vi "Hormiga_analogWrite.vi"(8 "error in (no error)":errorcluster, 9 "Analog Value":u16(slide) scale=0.0..1000.0, 10 "Terminal":u8=13, 11 "VISA Refnum in":refnum<visa-resource-name>) -> (0 "error out":errorcluster, 2 "Returned Value":u16, 3 "VISA Refnum out":refnum<visa-resource-name>)   [LabVIEW 2016]
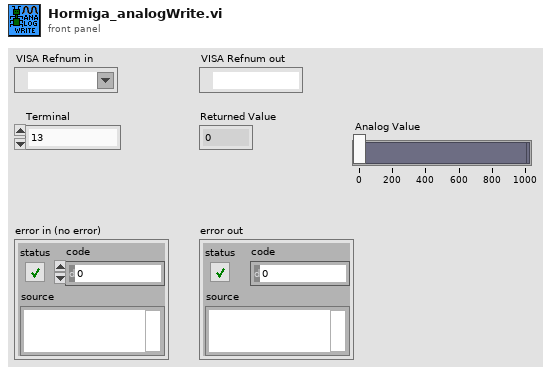
[diagram p1: front panel]
types:
  T1 = enum16{"pinMode", "digitalWrite", "digitalRead", "analogRead", "analogWrite"}
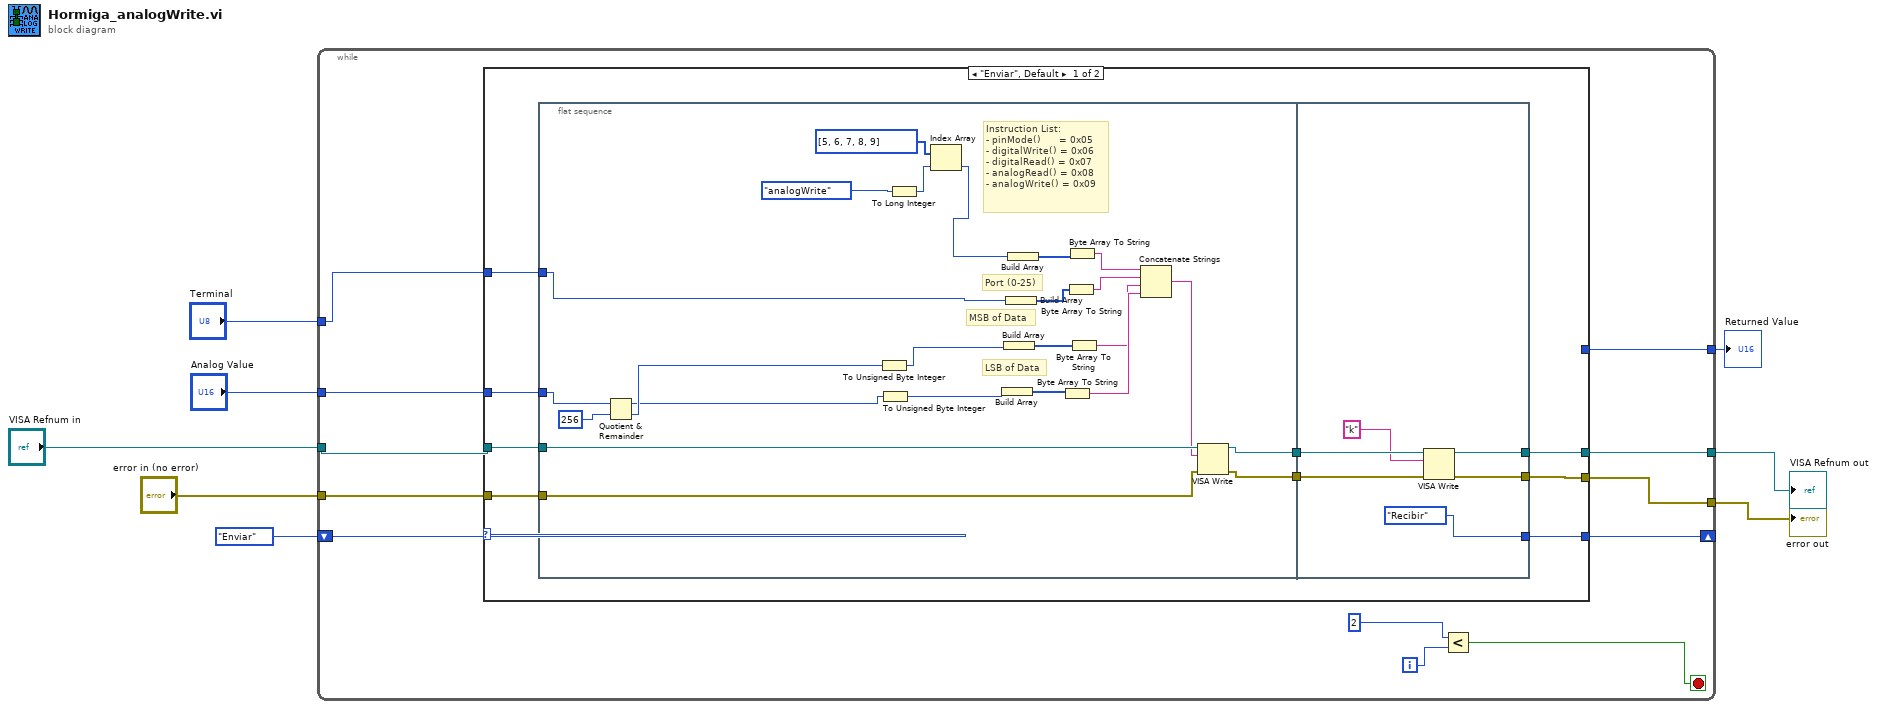
[diagram p0: block diagram]
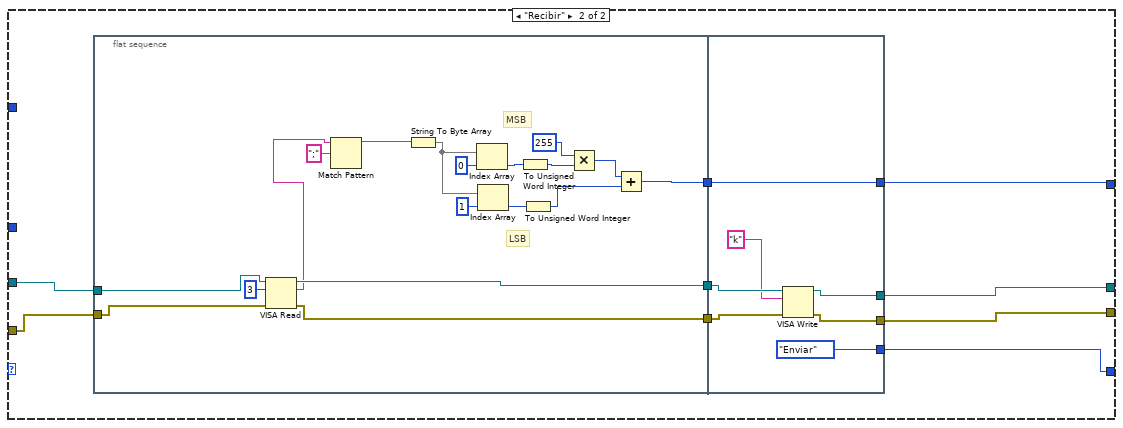
[diagram p2: hidden frame]
diagram:
  n1 = while {
    shift-right: [w15] -> _
    shift-left: enum16{"Enviar", "Recibir"}."Enviar" -> [w20]
    tunnel: "error in (no error)" -> [w19]
    tunnel: "VISA Refnum in" -> [w18]
    tunnel: [w17] -> w4
    tunnel: [w16] -> w5
    tunnel: "Terminal" -> [w11]
    tunnel: [w10] -> w8
    tunnel: "Analog Value" -> [w9]
    i -> [w13]
    stop <- w14 stop-if-true
    n2 = case shown="\"Enviar\", Default" w20 {
      tunnel: w19 -> [w29 w68]
      tunnel: w18 -> [w28 w67]
      tunnel: [w25 w64] -> w17
      tunnel: [w24 w63] -> w16
      tunnel: [w23 w62] -> w15
      tunnel: w11 -> [w22 _]
      tunnel: [_ w60] -> w10
      tunnel: w9 -> [w21 _]
      frame "Enviar", Default {
        n3 = flat-sequence {
          tunnel: w29 -> [w53]
          tunnel: w28 -> [w52]
          tunnel: [w51] -> w27
          tunnel: [w50] -> w26
          tunnel: w22 -> [w30]
          tunnel: w21 -> [w34]
          tunnel: w27 -> [w59]
          tunnel: w26 -> [w58]
          tunnel: [w56] -> w25
          tunnel: [w55] -> w24
          tunnel: [enum16{"Enviar", "Recibir"}."Recibir"] -> w23
          frame #0 {
            # "Instruction List:\n- pinMode()      = 0x05\n- digitalWrite() = 0x06\n- digitalRead() = 0x07\n- analogRead() = 0x08\n- analogWrite() = 0x09"
            # "LSB of Data"
            # "MSB of Data"
            # "Port (0-25)"
            n4 = Quotient & Remainder(x=w34, y=u16 256) -> (x-y*floor(x/y)=w31:u16, floor(x/y)=w32:u16)
            n5 = To Unsigned Byte Integer(number=w32) -> (unsigned 8bit integer=w35:u8)
            n6 = To Unsigned Byte Integer(number=w31) -> (unsigned 8bit integer=w36:u8)
            n7 = To Long Integer(number=T1."analogWrite") -> (32bit integer=w39:i32)
            n8 = Index Array(array=u8[] [5, 6, 7, 8, 9], index=w39) -> (element=w38:u8)
            n9 = Build Array(w36) -> (w46:u8[])
            n10 = Build Array(w35) -> (w47:u8[])
            n11 = Build Array(w30) -> (w48:u8[])
            n12 = Build Array(w38) -> (w49:u8[])
            n13 = Byte Array To String(unsigned byte array=w46) -> (string=w45:string)
            n14 = Byte Array To String(unsigned byte array=w48) -> (string=w43:string)
            n15 = Byte Array To String(unsigned byte array=w49) -> (string=w42:string)
            n16 = Byte Array To String(unsigned byte array=w47) -> (string=w44:string)
            n17 = Concatenate Strings(w42, w43, w44, w45) -> (w37:string)
            n18 = VISA Write(VISA resource name=w52, write buffer=w37, error in (no error)=w53) -> (VISA resource name out=w50:refnum<visa-resource-name>, error out=w51:errorcluster)  [unwired: 1 out]
          }
          frame #1 {
            n19 = VISA Write(VISA resource name=w58, write buffer="k", error in (no error)=w59) -> (VISA resource name out=w55:refnum<visa-resource-name>, error out=w56:errorcluster)  [unwired: 1 out]
          }
        }
      }
      frame "Recibir" {
        n20 = flat-sequence {
          tunnel: w68 -> [w70]
          tunnel: w67 -> [w69]
          tunnel: [w86] -> w66
          tunnel: [w85] -> w65
          tunnel: [w79] -> w61
          tunnel: w66 -> [w93]
          tunnel: w65 -> [w92]
          tunnel: [w90] -> w64
          tunnel: [w89] -> w63
          tunnel: [enum16{"Enviar", "Recibir"}."Enviar"] -> w62
          tunnel: w61 -> [w87]
          tunnel: [w87] -> w60
          frame #0 {
            # "MSB"
            # "LSB"
            n21 = VISA Read(VISA resource name=w69, byte count=u32 3, error in (no error)=w70) -> (VISA resource name out=w85:refnum<visa-resource-name>, read buffer=w76:string, error out=w86:errorcluster)  [unwired: 1 out]
            n22 = Match Pattern(string=w76, regular expression=";") -> (before substring=w78:string)  [unwired: 1 in, 3 out]
            n23 = String To Byte Array(string=w78) -> (unsigned byte array=w84:u8[])
            n24 = Index Array(array=w84, index=0) -> (element=w75:u8)
            n25 = Index Array(array=w84, index=1) -> (element=w73:u8)
            n26 = To Unsigned Word Integer(number=w75) -> (unsigned 16bit integer=w74:u16)
            n27 = To Unsigned Word Integer(number=w73) -> (unsigned 16bit integer=w72:u16)
            n28 = Multiply(x=u16 255, y=w74) -> (x*y=w81:u16)
            n29 = Add(x=w81, y=w72) -> (x+y=w79:u16)
          }
          frame #1 {
            n30 = VISA Write(VISA resource name=w92, write buffer="k", error in (no error)=w93) -> (VISA resource name out=w89:refnum<visa-resource-name>, error out=w90:errorcluster)  [unwired: 1 out]
          }
        }
      }
    }
    n31 = Less?(x=2, y=w13) -> (x < y?=w14:bool)
  }
  "Returned Value" <- w8
  "VISA Refnum out" <- w5
  "error out" <- w4
